vi "pain in.vi"() -> ()   [LabVIEW 2016]
panel:
  in  "Motor Name":string
  in  "Motor state":T1={"Statusword"=0, "Warnings"=16, "Error code"=16, "Error register"=8, "Controller temperature"=8, "Motor temperature"=8, "Troque actual value"=16, "Velocity actual value"=1617690656, "Electric power"=539230240, "DC current"=539164704, "Phase A current"=16, "Phase B current"=16, "Current demand"=16}
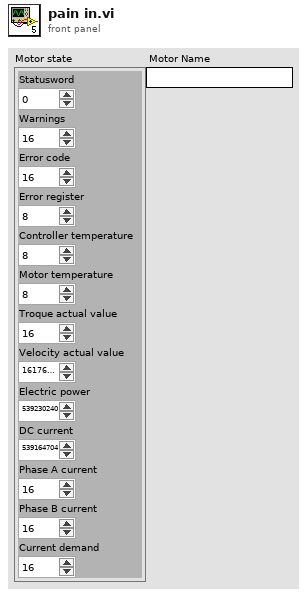
[diagram p1: front panel]
types:
  T1 = cluster{"Statusword":u16, "Warnings":u16, "Error code":u16, "Error register":u8, "Controller temperature":u8, "Motor temperature":u8, "Troque actual value":u16, "Velocity actual value":u32, "Electric power":u32, "DC current":u32, "Phase A current":u16, "Phase B current":u16, "Current demand":u16}
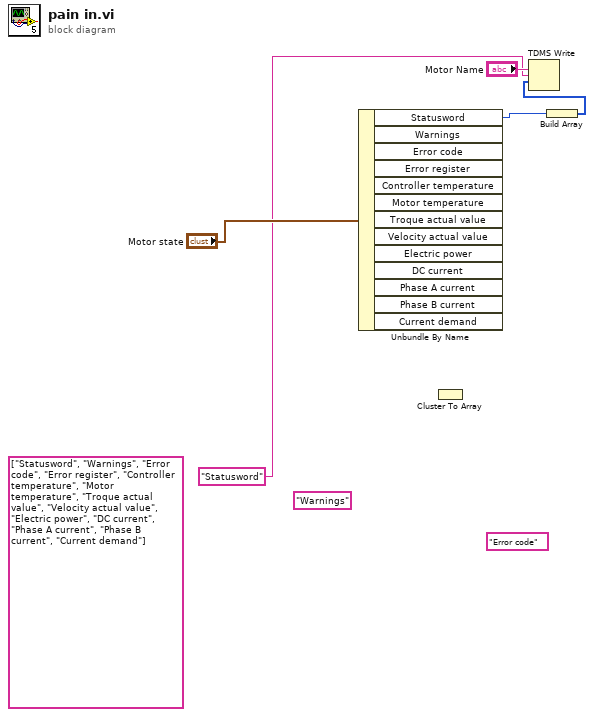
[diagram p0: block diagram]
diagram:
  (unwired) "Error code"
  (unwired) "Warnings"
  w5 = string[] ["Statusword", "Warnings", "Error code", "Error register", "Controller temperature", "Motor temperature", "Troque actual value", "Velocity actual value", "Electric power", "DC current", "Phase A current", "Phase B current", "Current demand"] ("channel name(s) in (Untitled)")
  n1 = Unbundle By Name("Motor state") -> ("Statusword"=w3:u16)  [unwired: 12 out]
  n2 = Cluster To Array() -> ()  [unwired: 1 in, 1 out]
  n3 = Build Array(w3) -> (w2:u16[])
  n4 = TDMS Write(5:"Motor Name", 7:"Statusword", 9:w2) -> ()  [unwired: 3 in, 4 out]
